vi "PadArray.vi"(8 "Pad Length":i32, 11 "Input Array":dbl[](array[numeric])) -> (3 "Padded Array":dbl[](array[numeric]))   [LabVIEW 2016]
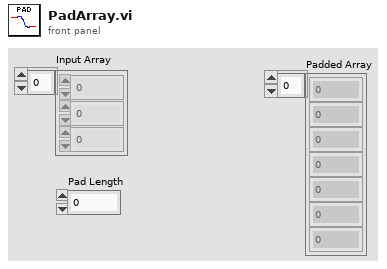
[diagram p1: front panel]
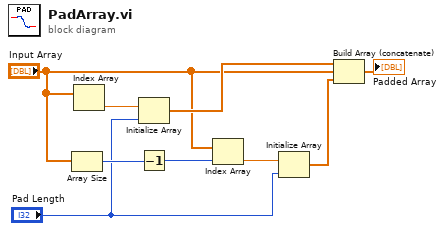
[diagram p0: block diagram]
diagram:
  n1 = Array Size(array="Input Array") -> (size(s)=w6:i32)
  n2 = Index Array(array="Input Array") -> (element=w9:dbl)  [unwired: 1 in]
  n3 = Initialize Array(w9, "Pad Length") -> (w8:dbl[])
  n4 = Decrement(x=w6) -> (x-1=w5:i32)
  n5 = Index Array(array="Input Array", index=w5) -> (element=w3:dbl)
  n6 = Initialize Array(w3, "Pad Length") -> (w1:dbl[])
  n7 = Build Array (concatenate)(w8, "Input Array", w1) -> (→"Padded Array":dbl[])
